vi "Initialize.vi"(8 "error in (no error)":errorcluster, 11 "SubPnl Refnum":refnum<vi>) -> (0 "error out":errorcluster, 3 "QTab Class out":refnum<class "QTab Class.lvclass">)   [LabVIEW 2020, in "QTab.lvlib" / "QTab Class.lvclass"]
uses:
  QTab Class.lvclass
  QTab Class.lvclass/QTab Class.ctl
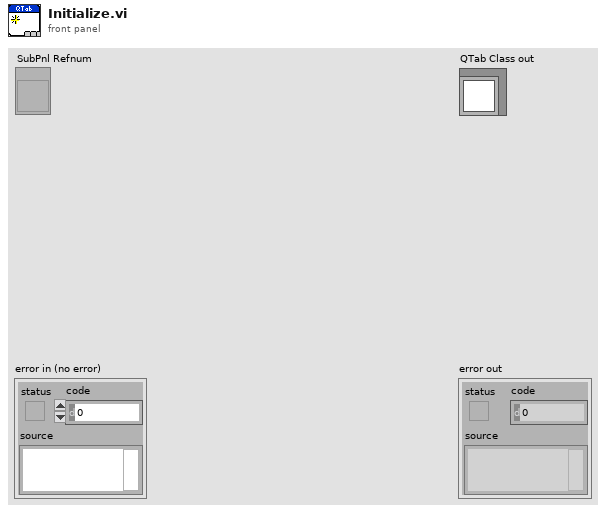
[diagram p1: front panel]
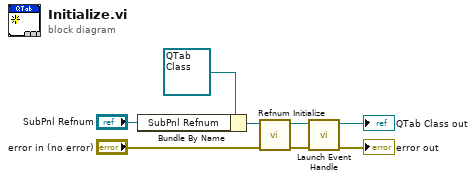
[diagram p0: block diagram]
diagram:
  n1 = Bundle By Name(cluster=refnum<class "QTab Class.lvclass"> refnum ("QTab Class out"), "SubPnl Refnum"="SubPnl Refnum") -> (w5:refnum<class "QTab Class.lvclass">)
  n2 = call "Refnum Initialize.vi"("error in (no error)"="error in (no error)", "QTab Class in"=w5) -> ("error out"=w3:errorcluster, "QTab Class out"=w4:refnum<class "QTab Class.lvclass">)  [unwired: 8 in]
  n3 = call "Launch Event Handle.vi"("error in (no error)"=w3, "QTab Class in"=w4) -> ("error out"=→"error out":errorcluster, "QTab Class out"=→"QTab Class out":refnum<class "QTab Class.lvclass">)  [unwired: 8 in]
